vi "Set Dialog Properties.vi"(8 "Error In (no error)":errorcluster, 10 "Enable Dialog Properties":bool, 11 "VI Ref In":refnum<vi>) -> (0 "Error Out":errorcluster, 3 "VI Ref Out":refnum<vi>)   [LabVIEW 2012]
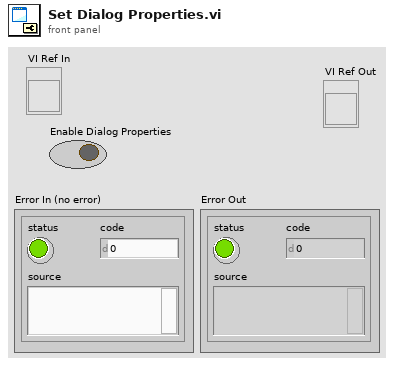
[diagram p1: front panel]
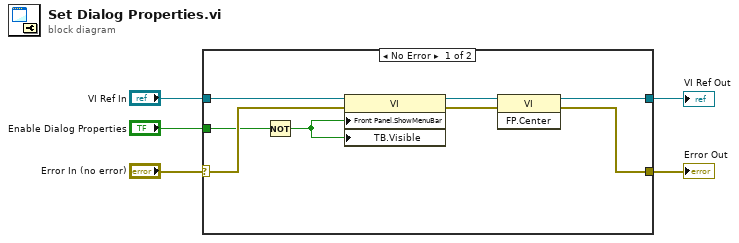
[diagram p0: block diagram]
diagram:
  n1 = case shown="No Error" "Error In (no error)" {
    selector: "Error In (no error)" -> [w10 w15]
    tunnel: "Enable Dialog Properties" -> [w7 _]
    tunnel: "VI Ref In" -> [w11 w14]
    tunnel: [w9 w14] -> w1
    tunnel: [w8 w15] -> w2
    frame No Error {
      n2 = Not(x=w7) -> (.not. x?=w6:bool)
      n3 = property class="VI"(reference=w11, error in=w10, "Front Panel.ShowMenuBar"=w6, "TB.Visible"=w6) -> (reference out=w12:refnum<vi>, error out=w13:errorcluster)
      n4 = invoke class="VI" method="FP.Center"(reference=w12, error in=w13) -> (reference out=w9:refnum<vi>, error out=w8:errorcluster)  [unwired: 1 in, 1 out]
    }
    frame Error {
    }
  }
  "Error Out" <- w2
  "VI Ref Out" <- w1
